vi "Set DDS.vi"(0 "NMR in":refnum<class "NMR.lvclass">, 5 "Power Level":u16=512 max=1023 step=1, 7 "Phase":u16=180 max=270 step=90, 9 "Frequency":dbl=8000000.0 min=1.0 format="%^#_6e", 11 "error in (no error)":errorcluster) -> (4 "NMR out":refnum<class "NMR.lvclass">, 10 "String as ASCII":string, 15 "error out":errorcluster)   [LabVIEW 2011, in "NMR.lvclass"]
uses:
  NMR.lvclass
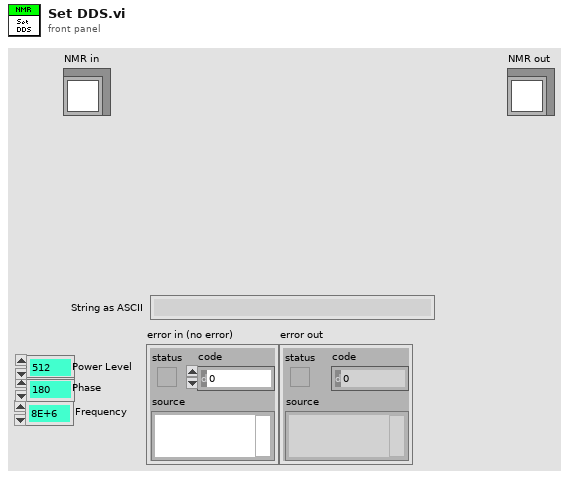
[diagram p1: front panel]
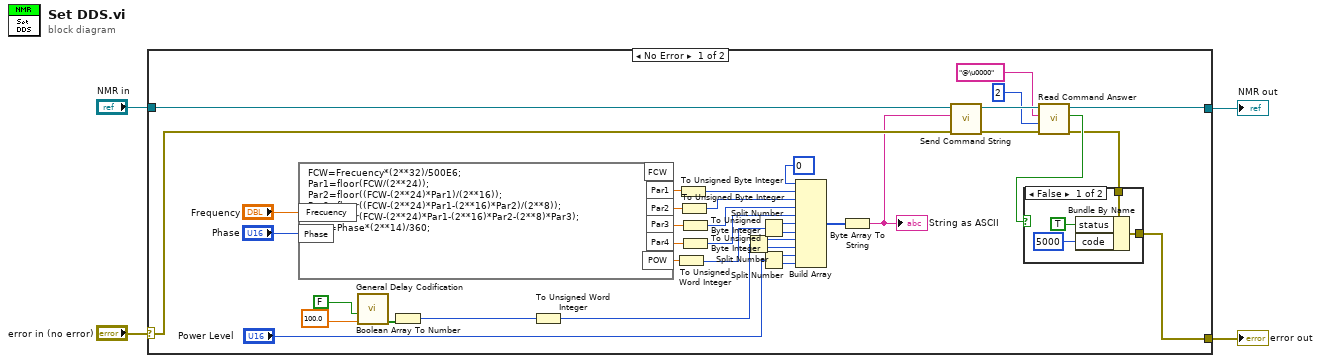
[diagram p0: block diagram]
diagram:
  n1 = case shown="No Error" "error in (no error)" {
    selector: "error in (no error)" -> [w38 w48]
    tunnel: [w10 w48] -> w3
    tunnel: [w39 w47] -> w1
    tunnel: "NMR in" -> [w41 w47]
    frame No Error {
      n2 = formula code="FCW=Frecuency*(2**32)/500E6;\nPar1=floor(FCW/(2**24));\nPar2=floor((FCW-(2**24)*Par1)/(2**16));\nPar3=floor((FCW-(2**24)*Par1-(2**16)*Par2)/(2**8));\nPar4=floor(FCW-(2**24)*Par1-(2**16)*Par2-(2**8)*Par3);\nPOW=Phase*(2**14)/360;"("Frecuency"="Frequency", "Phase"="Phase") -> ("Par1"=w31:dbl, "Par2"=w32:dbl, "Par3"=w33:dbl, "Par4"=w34:dbl, "POW"=w35:dbl)  [unwired: 1 out]
      n3 = call "General Delay Codification.vi"("Delay"=100.0, "ms/us Delay"=FALSE) -> ("Final array"=w9:bool[])  [unwired: 8 in, 1 out]
      n4 = Boolean Array To Number(Boolean array=w9) -> (number=w5:u32)
      n5 = To Unsigned Word Integer(number=w5) -> (unsigned 16bit integer=w6:u16)
      n6 = To Unsigned Word Integer(number=w35) -> (unsigned 16bit integer=w23:u16)
      n7 = To Unsigned Byte Integer(number=w31) -> (unsigned 8bit integer=w27:u8)
      n8 = To Unsigned Byte Integer(number=w32) -> (unsigned 8bit integer=w26:u8)
      n9 = To Unsigned Byte Integer(number=w33) -> (unsigned 8bit integer=w25:u8)
      n10 = To Unsigned Byte Integer(number=w34) -> (unsigned 8bit integer=w24:u8)
      n11 = Split Number(x=w6) -> (hi(x)=w20:u8, lo(x)=w19:u8)
      n12 = Split Number(x=w23) -> (hi(x)=w22:u8, lo(x)=w21:u8)
      n13 = Split Number(x="Power Level") -> (hi(x)=w17:u8, lo(x)=w16:u8)
      n14 = Build Array(u32 0 ("element"), w27, w26, w25, w24, w22, w21, w20, w19, w17, w16) -> (w36:u32[])
      n15 = Byte Array To String(unsigned byte array=w36) -> (string=w15:string)
      "String as ASCII" <- w15
      n16 = call-dynamic "Send Command String.vi"("error in (no error)"=w38, "Command String"=w15, "NMR in"=w41) -> ("error out"=w37:errorcluster, "NMR out"=w40:refnum<class "NMR.lvclass">)  [unwired: 7 in]
      n17 = call-dynamic "Read Command Answer.vi"("error in (no error)"=w37, "bytes to read"=u32 2 ("Number bytes Read"), "String Seached"="@\u0000" ("search char"), "NMR in"=w40) -> ("error out"=w11:errorcluster, "Expected Answer?"=w12:bool, "NMR out"=w39:refnum<class "NMR.lvclass">)  [unwired: 5 in]
      n18 = case shown="False" w12 {
        tunnel: w11 -> [w43 w46]
        tunnel: [w42 w46] -> w10
        frame False {
          n19 = Bundle By Name(cluster=w43, "status"=TRUE, "code"=5000) -> (w42:errorcluster)
        }
        frame True {
        }
      }
    }
    frame Error {
    }
  }
  "error out" <- w3
  "NMR out" <- w1
